vi "Test MQTT-1.5.3-1.vi"(8 "error in (no error)":errorcluster) -> (0 "error out":errorcluster)   [LabVIEW 2013]
uses:
  <vilib>/addons/_JKI Toolkits/Caraya/classes/Test/Test.lvclass
  <vilib>/addons/_JKI Toolkits/Caraya/classes/Assert/Assert.lvclass
  <vilib>/LabVIEW Open Source Project/MQTT Control Packets/Control Packets/ControlPacket/ControlPacket.lvclass
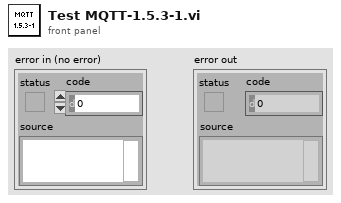
[diagram p1: front panel]
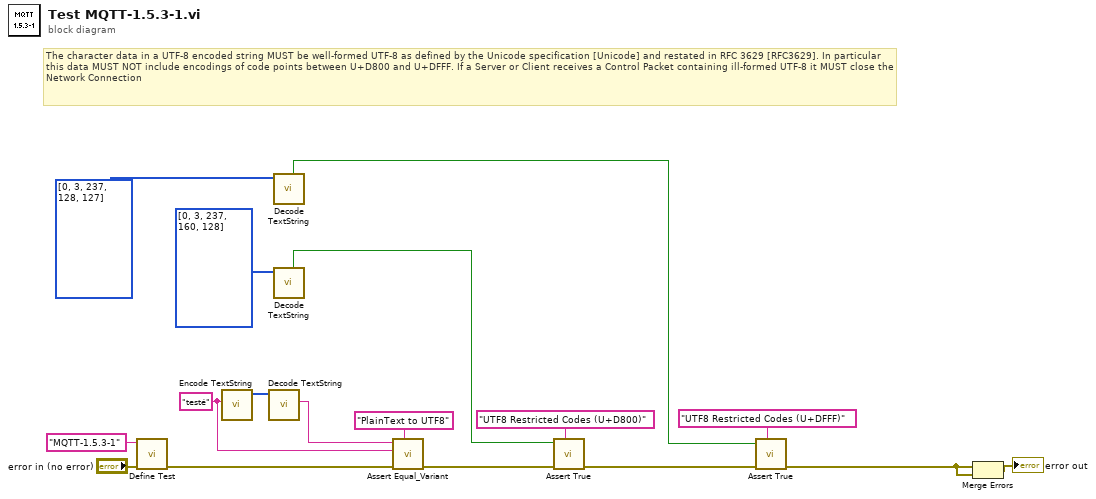
[diagram p0: block diagram]
diagram:
  w12 = "testé" ("Text String")
  # "The character data in a UTF-8 encoded string MUST be well-formed UTF-8 as defined by the Unicode specification [Unicode] and restated in RFC 3629 [RFC3629]. In particular this data MUST NOT include encodings of code points between U+D800 and U+DFFF. If a Server or Client receives a Control Packet containing ill-formed UTF-8 it MUST close the Network Connection"
  n1 = call <vilib>:"Define Test.vi"("error in (no error)"="error in (no error)", "Label (VI Title)"="MQTT-1.5.3-1") -> ("error out"=w16:errorcluster)  [unwired: 9 in]
  n2 = call <vilib>:"Encode TextString.vi"("Text String"=w12) -> ("Length-Prefixed Field"=w10:u8[])  [unwired: 10 in]
  n3 = call <vilib>:"Decode TextString.vi"("Length-Prefixed Field"=w10) -> ("Text String"=w13:string)  [unwired: 8 in, 2 out]
  n4 = call <vilib>:"Decode TextString.vi"("Length-Prefixed Field"=u8[] [0, 3, 237, 128, 127]) -> ("restricted code"=w1:bool)  [unwired: 8 in, 2 out]
  n5 = call <vilib>:"Decode TextString.vi"("Length-Prefixed Field"=u8[] [0, 3, 237, 160, 128]) -> ("restricted code"=w6:bool)  [unwired: 8 in, 2 out]
  n6 = call <vilib>:"Assert Equal_Variant.vi"("Label"="PlainText to UTF8", "error in (no error)"=w16, "Y"=w12, "X"=w13) -> ("error out"=w7:errorcluster)  [unwired: 7 in]
  n7 = call <vilib>:"Assert True.vi"("Label"="UTF8 Restricted Codes (U+D800)", "error in (no error)"=w7, "True?"=w6) -> ("error out"=w3:errorcluster)  [unwired: 8 in]
  n8 = call <vilib>:"Assert True.vi"("Label"="UTF8 Restricted Codes (U+DFFF)", "error in (no error)"=w3, "True?"=w1) -> ("error out"=w2:errorcluster)  [unwired: 8 in]
  n9 = Merge Errors(w2, w2) -> (→"error out":errorcluster)
